vi "Span Register setzen.vi"(6 "init":bool, 8 "error in (no error)":errorcluster caption="Fehler (Eingang, kein Fehler)", 10 "GD Span Eingänge":refnum<vi>, 11 "automatisch Boolesch (Eingang)":refnum<vi>) -> (0 "error out":errorcluster caption="Fehler (Ausgang)", 1 "Anzahl Span out":i32, 2 "GD Span Eingänge out":refnum<vi>, 3 "automatisch Boolesch (Ausgang)":refnum<vi>, 4 "automatisch out":T1, 5 "auto Deaktiviert":T2(ring), 7 "GD Span Eingänge":u16)   [LabVIEW 2020, in "Linearisierung v2.lvlib" / "SpanEinstellungen.lvlib"]
uses:
  SpanEinstellungen.lvlib
  Seiten/System Einstellungen V2/Konfig Gasflasche.ctl
  Aktion FGV SpanEinstellungen.ctl
  Visualisierungs Elemente/String - Eingabefeld.ctl
  Seiten/System Einstellungen V2/System Einstellungen V2.lvlib
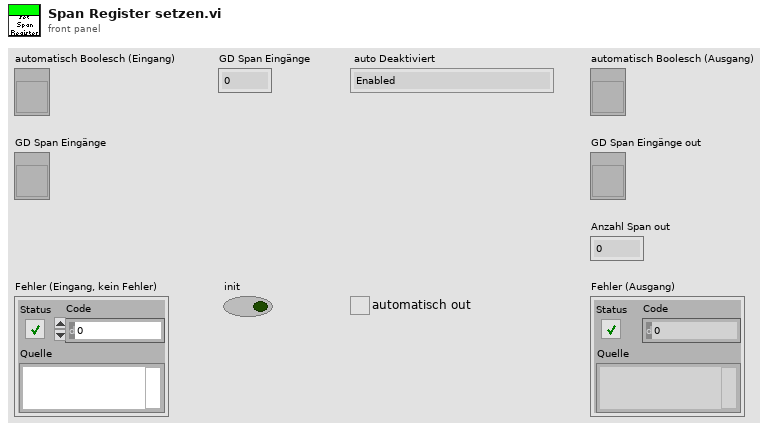
[diagram p1: front panel]
types:
  T1 = typedef "System Einstellungen V2.lvlib/Konfig Gasflasche.ctl" = bool
  T2 = enum8{"Enabled", "Disabled", "Disabled and Grayed Out"}
  T3 = typedef "Linearisierung v2.lvlib/SpanEinstellungen.lvlib/Aktion FGV SpanEinstellungen.ctl" = enum16{"lesen", "schreiben", "laden", "speichern", "RegisterRef", "automatisch", "init", "PDF Params", "Punkte umkehren"}
  T4 = cluster{"HauptRegister in":refnum<vi>, "SpanRegister in":refnum<vi>}
  T5 = typedef "String - Eingabefeld.ctl" = string
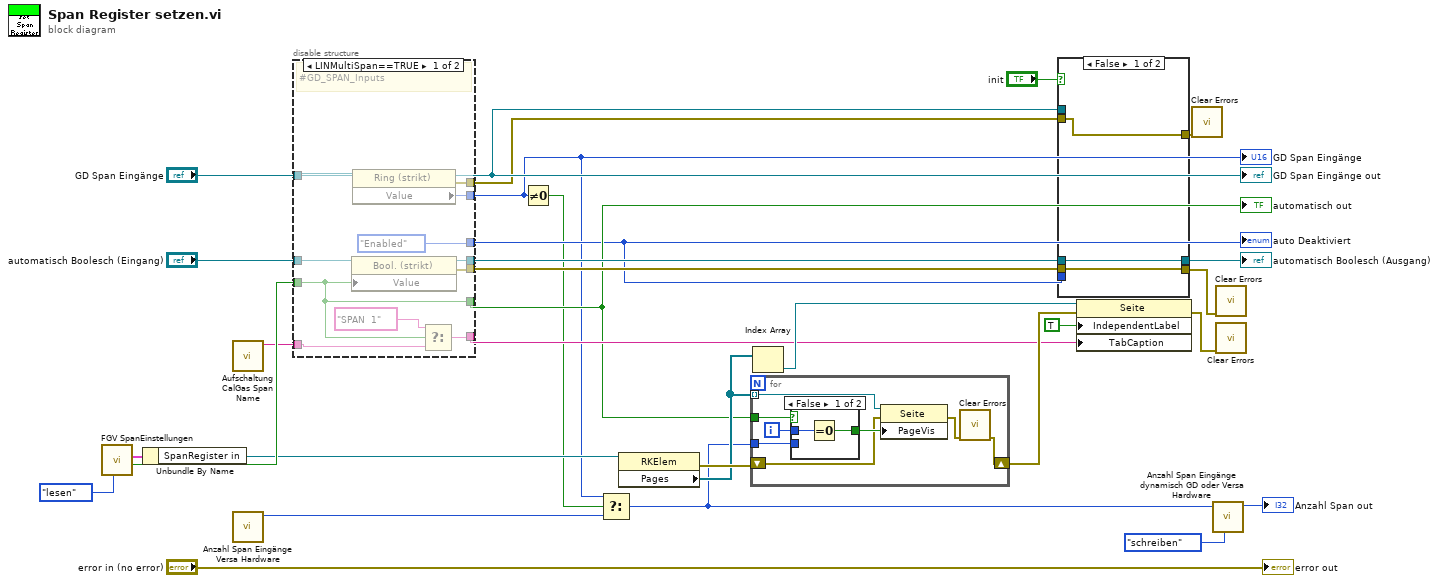
[diagram p0: block diagram]
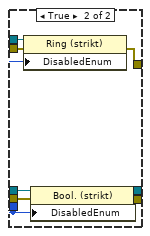
[diagram p2: hidden frame]
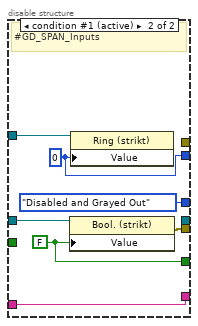
[diagram p3: hidden frame]
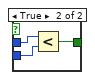
[diagram p4: hidden frame]
diagram:
  n1 = call "FGV SpanEinstellungen.vi"("Aktion"=Aktion_FGV_SpanEinstellungen."lesen") -> ("automatisch out"=w26:T1, "RegisterRefs out"=w20:T4)  [unwired: 6 in, 3 out]
  n2 = Unbundle By Name(w20) -> ("SpanRegister in"=w12:refnum<vi>)
  n3 = call "Aufschaltung CalGas Span Name.vi"() -> ("Span Name"=w21:T5)  [unwired: 11 in]
  n4 = call "Anzahl Span Eingänge Versa Hardware.vi"() -> ("Anzahl Span"=w3:i32)  [unwired: 11 in]
  n5 = disable-structure shown="LINMultiSpan==TRUE" {
    disable-tunnel: [T2."Enabled" ("Deaktiviert") T2."Disabled and Grayed Out" ("Deaktiviert")] -> w11
    disable-tunnel: w26 -> [w38 _]
    disable-tunnel: [w35 w44] -> w15
    disable-tunnel: [w38 w47] -> w13
    disable-tunnel: "automatisch Boolesch (Eingang)" -> [w40 w45]
    disable-tunnel: [w39 w46] -> w22
    disable-tunnel: w21 -> [w37 w44]
    disable-tunnel: [w34 _] -> w17
    disable-tunnel: "GD Span Eingänge" -> [w33 w43]
    disable-tunnel: [w32 _] -> w8
    disable-tunnel: [w31 w42] -> w6
    frame condition #0 {
      # "#GD_SPAN_Inputs"
      n6 = property class="Bool. (strikt)"(reference=w40, "Value"=w38) -> (reference out=w34:refnum<vi>, error out=w39:errorcluster)  [unwired: 1 in]
      n7 = property class="Ring (strikt)"(reference=w33) -> (error out=w32:errorcluster, "Value"=w31:u16)  [unwired: 1 in, 1 out]
      n8 = Select(t=T5 "SPAN  1" ("Span Name"), s=w38, f=w37) -> (s? t:f=w35:T5)
    }
    frame condition #1 (active) {
      w42 = u16 0 ("Wert")
      w47 = FALSE
      # "#GD_SPAN_Inputs"
      n9 = property class="Bool. (strikt)"(reference=w45, "Value"=w47) -> (error out=w46:errorcluster)  [unwired: 1 in, 1 out]
      n10 = property class="Ring (strikt)"(reference=w43, "Value"=w42) -> ()  [unwired: 1 in, 2 out]
    }
  }
  "auto Deaktiviert" <- w11
  "automatisch out" <- w13
  "GD Span Eingänge" <- w6
  n11 = Not Equal To 0?(x=w6) -> (x != 0?=w7:bool)
  n12 = Select(t=w6, s=w7, f=w3) -> (s? t:f=w2:i32)
  n13 = property class="RKElem"(reference=w12) -> (error out=w24:errorcluster, "Pages"=w19:refnum<vi>[])  [unwired: 1 in, 1 out]
  n14 = for {
    tunnel: w19 -> [w56] mode=indexing
    tunnel: w13 -> [w52]
    tunnel: w2 -> [w51]
    shift-right: [w49] -> w23
    shift-left: w24 -> [w50]
    i -> [w54]
    n15 = case shown="False" w52 {
      tunnel: w54 -> [w58 w60]
      tunnel: [w57 w61] -> w53
      tunnel: w51 -> [_ w59]
      frame False {
        n16 = Equal To 0?(x=w58) -> (x = 0?=w57:bool)
      }
      frame True {
        n17 = Less?(x=w60, y=w59) -> (x < y?=w61:bool)
      }
    }
    n18 = property class="Seite"(reference=w56, error in=w50, "PageVis"=w53) -> (error out=w55:errorcluster)  [unwired: 1 out]
    n19 = call <vilib>:"Clear Errors.vi"("error in (no error)"=w55) -> ("error out"=w49:errorcluster)  [unwired: 5 in, 1 out]
  }
  n20 = Index Array(array=w19) -> (element=w29:refnum<vi>)  [unwired: 1 in]
  n21 = case shown="False" "init" {
    tunnel: [w63 w72] -> w28
    tunnel: w22 -> [w63 w71]
    tunnel: w17 -> [w62 w70]
    tunnel: [w62 w69] -> w16
    tunnel: w11 -> [_ w68]
    tunnel: "GD Span Eingänge" -> [_ w67]
    tunnel: [w64 w66] -> w9
    tunnel: w8 -> [w64 w65]
    frame False {
    }
    frame True {
      n22 = property on="Eigenschaftsknoten" class="Ring (strikt)"(reference=w67, error in=w65, "DisabledEnum"=w68) -> (error out=w66:errorcluster)  [unwired: 1 out]
      n23 = property on="Eigenschaftsknoten" class="Bool. (strikt)"(reference=w70, error in=w71, "DisabledEnum"=w68) -> (reference out=w69:refnum<vi>, error out=w72:errorcluster)
    }
  }
  "automatisch Boolesch (Ausgang)" <- w16
  n24 = property class="Seite"(reference=w29, error in=w23, "IndependentLabel"=TRUE ("Unabhängige Beschriftung"), "TabCaption"=w15) -> (error out=w30:errorcluster)  [unwired: 1 out]
  n25 = call <vilib>:"Clear Errors.vi"("error in (no error)"=w9) -> ()  [unwired: 5 in, 2 out]
  n26 = call "Anzahl Span Eingänge dynamisch GD oder Versa Hardware.vi"("Aktion"=enum16{"lesen", "schreiben"}."schreiben", "Anzahl Span in"=w2) -> ("Anzahl Span out"=→"Anzahl Span out":i32)  [unwired: 9 in]
  n27 = call <vilib>:"Clear Errors.vi"("error in (no error)"=w28) -> ()  [unwired: 5 in, 2 out]
  n28 = call <vilib>:"Clear Errors.vi"("error in (no error)"=w30) -> ()  [unwired: 5 in, 2 out]
  "error out" <- "error in (no error)"
  "GD Span Eingänge out" <- "GD Span Eingänge"
